vi "mod_IQ Impairments Quadrature Skew.vi"(0 "Input Complex Waveform":T1 {"Y" format="%.3f"; "dt" format="%^.2e"; "t0" format="%.4f"}, 2 "Quadrature Skew, deg":dbl format="%.2f", 11 "error in (no error)":errorcluster) -> (4 "Output Complex Waveform":T1 {"Y" format="%.3f"; "dt" format="%^.2e"; "t0" format="%.4f"}, 15 "error out":errorcluster)   [LabVIEW 2020, in "niDMT.lvlib"]
doc: "Performs the Quadrature Skew operation for IQ Impairment of an Input Data Waveform."
uses:
  <vilib>/addons/Modulation/niDMT.lvlib
  <vilib>/addons/Modulation/Analog/controls/Complex Data Waveform.ctl
  <vilib>/addons/Modulation/niAMT.lvlib
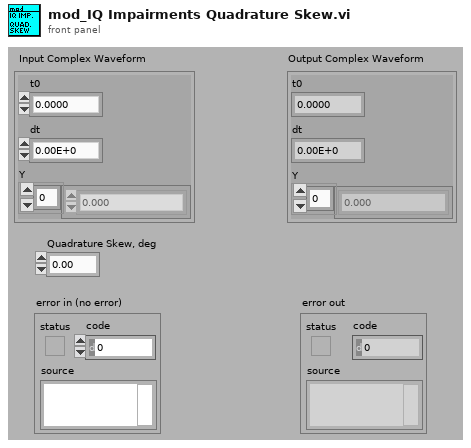
[diagram p1: front panel]
types:
  T1 = typedef "niAMT.lvlib/Complex Data Waveform.ctl" = cluster{"t0":dbl, "dt":dbl, "Y":cdb[]}
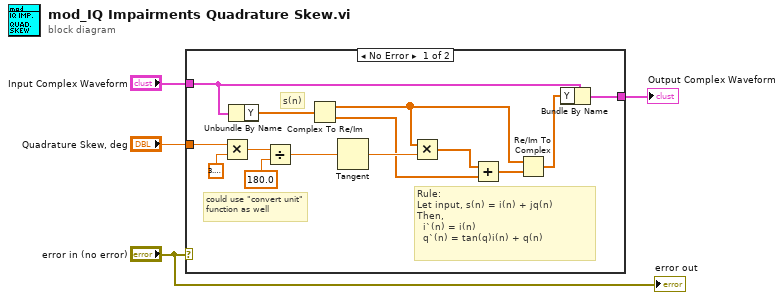
[diagram p0: block diagram]
diagram:
  n1 = case shown="No Error" "error in (no error)" {
    tunnel: "Quadrature Skew, deg" -> [w6 _]
    tunnel: "Input Complex Waveform" -> [w17 w19]
    tunnel: [w16 w19] -> w1
    frame No Error {
      # "s(n)"
      # "Rule:\nLet input, s(n) = i(n) + jq(n)\nThen,\n  i`(n) = i(n)\n  q`(n) = tan(q)i(n) + q(n)"
      # "could use \"convert unit\" function as well"
      n2 = Multiply(x=w6, y=3.141592653589793) -> (x*y=w14:dbl)
      n3 = Unbundle By Name(w17) -> ("Y"=w18:cdb[])
      n4 = Divide(x=w14, y=180.0) -> (x/y=w8:dbl)
      n5 = Complex To Re/Im(x + iy=w18) -> (x=w11:dbl[], y=w5:dbl[])
      n6 = Tangent(1:w8) -> (0:w7:dbl)
      n7 = Multiply(x=w11, y=w7) -> (x*y=w10:dbl[])
      n8 = Add(x=w10, y=w5) -> (x+y=w9:dbl[])
      n9 = Re/Im To Complex(1:w9, 2:w11) -> (0:w15:cdb[])
      n10 = Bundle By Name(cluster=w17, "Y"=w15) -> (w16:T1)
    }
    frame Error {
    }
  }
  "Output Complex Waveform" <- w1
  "error out" <- "error in (no error)"
